vi "ConfigSMU2ch_current.vi"(0 "IVI Refnum in":refnum<k15>, 1 "Channel DxSupply":string="0", 2 "Current Level DxSupply":dbl, 3 "Voltage Limit DxSupply":dbl, 11 "error in (no error)":errorcluster, 12 "Channel DxBoot0":string="0", 13 "Current Level DxBoot0":dbl, 14 "Voltage Limit DxBoot0":dbl) -> (4 "IVI Refnum out":refnum<k15>, 15 "error out":errorcluster)   [LabVIEW 2018]
uses:
  <instrlib>/niDCPower/nidcpower.llb/niDCPower Output Function.ctl
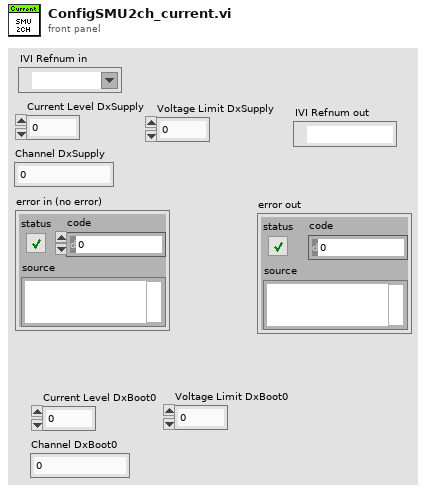
[diagram p1: front panel]
types:
  T1 = typedef "niDCPower Output Function.ctl" = i32
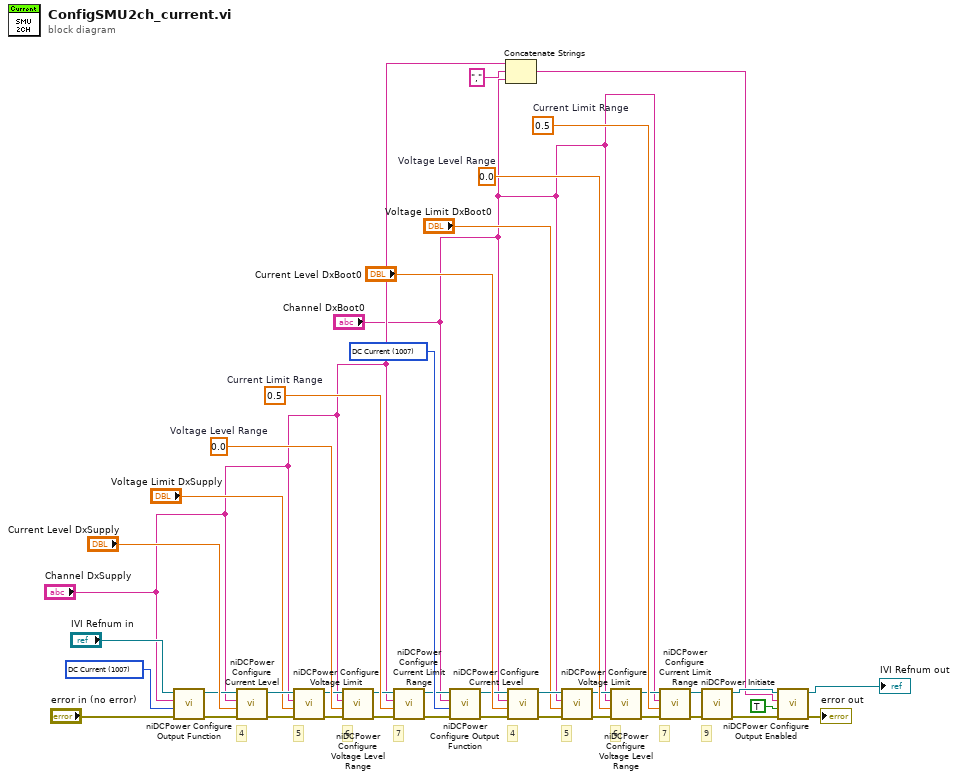
[diagram p0: block diagram]
diagram:
  w14 = T1 1007 items=["DC Voltage"=1006, "DC Current"=1007, "Pulse Voltage"=1049, "Pulse Current"=1050] ("output function")
  w23 = 0.0  # Voltage Level Range
  w24 = 0.5  # Current Limit Range
  w31 = T1 1007 items=["DC Voltage"=1006, "DC Current"=1007, "Pulse Voltage"=1049, "Pulse Current"=1050] ("output function")
  w40 = 0.0  # Voltage Level Range
  w41 = 0.5  # Current Limit Range
  # "7"
  # "6"
  # "5"
  # "4"
  # "9"
  # "7"
  # "6"
  # "5"
  # "4"
  n1 = call <instrlib>:"niDCPower Configure Output Function.vi"("error in (no error)"="error in (no error)", "output function"=w31, "channel name"="Channel DxSupply", "instrument handle"="IVI Refnum in") -> ("error out"=w30:errorcluster, "instrument handle out"=w29:refnum<k15>)  [unwired: 6 out]
  n2 = call <instrlib>:"niDCPower Configure Current Level.vi"("error in (no error)"=w30, "current level"="Current Level DxSupply", "channel name"="Channel DxSupply", "instrument handle"=w29) -> ("error out"=w33:errorcluster, "instrument handle out"=w34:refnum<k15>)  [unwired: 6 in]
  n3 = call <instrlib>:"niDCPower Configure Voltage Limit.vi"("error in (no error)"=w33, "voltage limit"="Voltage Limit DxSupply", "channel name"="Channel DxSupply", "instrument handle"=w34) -> ("error out"=w35:errorcluster, "instrument handle out"=w36:refnum<k15>)  [unwired: 6 in]
  n4 = call <instrlib>:"niDCPower Configure Voltage Level Range.vi"("error in (no error)"=w35, "voltage level range"=w40, "channel name"="Channel DxSupply", "instrument handle"=w36) -> ("error out"=w38:errorcluster, "instrument handle out"=w39:refnum<k15>)  [unwired: 6 out]
  n5 = call <instrlib>:"niDCPower Configure Current Limit Range.vi"("error in (no error)"=w38, "current limit range"=w41, "channel name"="Channel DxSupply", "instrument handle"=w39) -> ("error out"=w11:errorcluster, "instrument handle out"=w10:refnum<k15>)  [unwired: 6 out]
  n6 = call <instrlib>:"niDCPower Configure Output Function.vi"("error in (no error)"=w11, "output function"=w14, "channel name"="Channel DxBoot0", "instrument handle"=w10) -> ("error out"=w13:errorcluster, "instrument handle out"=w12:refnum<k15>)  [unwired: 6 out]
  n7 = Concatenate Strings("Channel DxSupply", "," ("string"), "Channel DxBoot0") -> (w3:string)
  n8 = call <instrlib>:"niDCPower Configure Current Level.vi"("error in (no error)"=w13, "current level"="Current Level DxBoot0", "channel name"="Channel DxBoot0", "instrument handle"=w12) -> ("error out"=w16:errorcluster, "instrument handle out"=w17:refnum<k15>)  [unwired: 6 in]
  n9 = call <instrlib>:"niDCPower Configure Voltage Limit.vi"("error in (no error)"=w16, "voltage limit"="Voltage Limit DxBoot0", "channel name"="Channel DxBoot0", "instrument handle"=w17) -> ("error out"=w18:errorcluster, "instrument handle out"=w19:refnum<k15>)  [unwired: 6 in]
  n10 = call <instrlib>:"niDCPower Configure Voltage Level Range.vi"("error in (no error)"=w18, "voltage level range"=w23, "channel name"="Channel DxBoot0", "instrument handle"=w19) -> ("error out"=w21:errorcluster, "instrument handle out"=w22:refnum<k15>)  [unwired: 6 out]
  n11 = call <instrlib>:"niDCPower Configure Current Limit Range.vi"("error in (no error)"=w21, "current limit range"=w24, "channel name"="Channel DxBoot0", "instrument handle"=w22) -> ("error out"=w1:errorcluster, "instrument handle out"=w2:refnum<k15>)  [unwired: 6 out]
  n12 = call <instrlib>:"niDCPower Initiate.vi"("error in (no error)"=w1, "instrument handle"=w2) -> ("error out"=w5:errorcluster, "instrument handle out"=w7:refnum<k15>)  [unwired: 2 in, 6 out]
  n13 = call <instrlib>:"niDCPower Configure Output Enabled.vi"("error in (no error)"=w5, "output enabled"=TRUE, "channel name"=w3, "instrument handle"=w7) -> ("error out"=→"error out":errorcluster, "instrument handle out"=→"IVI Refnum out":refnum<k15>)  [unwired: 6 in]
